vi "Init Logging.vi"(8 "error in":errorcluster, 10 "Handlers":refnum<class "Handler.lvclass">[](array[class]), 11 "Name":string) -> (0 "error out":errorcluster)   [LabVIEW 2024, in "hse-logger.lvlib"]
doc: "Initiates the *Simple Logging API*. A new logger object with the specified name and handlers is created and a reference (DVR) to this object is stored in a private FGV. All other functions from the *Simple Logging API* accessing this FGV to retrieve the logger object.\n\n____\nHAMPEL SOFTWARE ENGINEERING v2.2.2 (2025-01-16 15:41)"
uses:
  <vilib>/Hampel Software Engineering/HSE Logger/hse-logger.lvlib
  <vilib>/Hampel Software Engineering/HSE Logger/Handler/Handler.lvclass
  <vilib>/Hampel Software Engineering/HSE Logger/FGV Actions.ctl
  <vilib>/Hampel Software Engineering/HSE Logger/Logger/Logger.lvclass
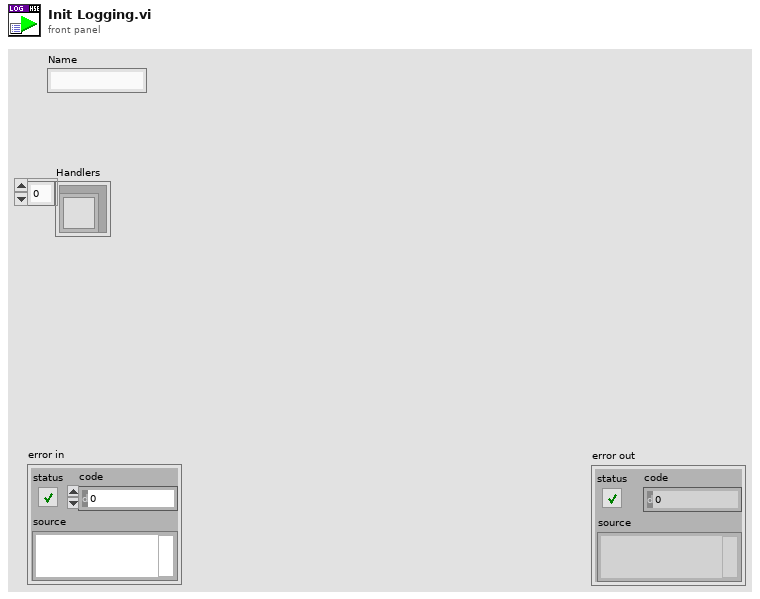
[diagram p1: front panel]
types:
  T1 = typedef "hse-logger.lvlib/FGV Actions.ctl" = enum16{"Set", "Get"}
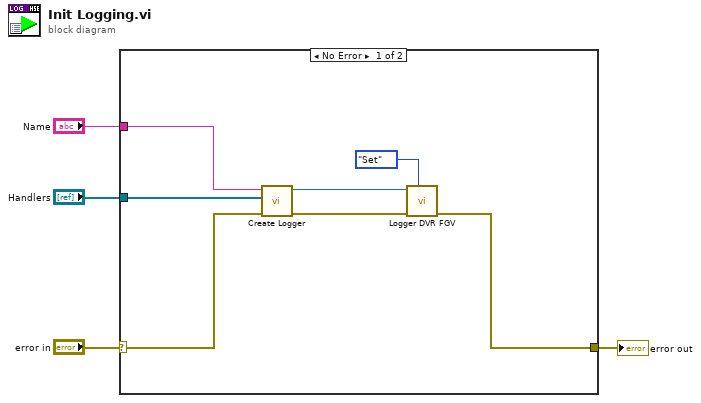
[diagram p0: block diagram]
diagram:
  n1 = case shown="No Error" "error in" {
    selector: "error in" -> [w10 w12]
    tunnel: [w6 w12] -> w3
    tunnel: "Name" -> [w11 _]
    tunnel: "Handlers" -> [w9 _]
    frame No Error {
      n2 = call <vilib>:"Create Logger.vi"("error in"=w10, "Handlers"=w9, "Name"=w11) -> ("error out"=w8:errorcluster, "Logger out"=w7:refnum<class "Logger.lvclass">)  [unwired: 7 in]
      n3 = call <vilib>:"Logger DVR FGV.vi"("FGV Actions"=FGV_Actions."Set", "error in"=w8, "Logger in"=w7) -> ("error out"=w6:errorcluster)  [unwired: 7 in, 1 out]
    }
    frame Error {
    }
  }
  "error out" <- w3
